vi "SGL to String Exchange.vi"(2 "SGL In":sgl, 3 "4字节字符串":string="C{™š") -> (0 "4字节字符串":string, 1 "IEE754Floatout":sgl format="%#_5f")   [LabVIEW 2015]
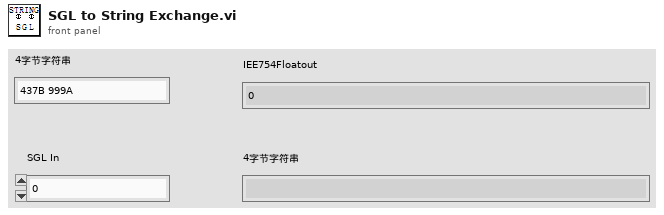
[diagram p1: front panel]
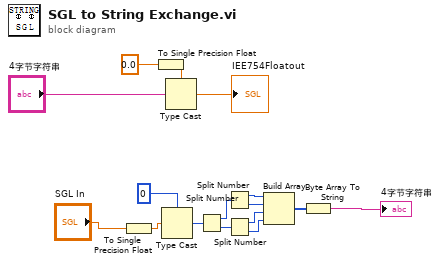
[diagram p0: block diagram]
diagram:
  n1 = To Single Precision Float(number="SGL In") -> (single precision float=w1:sgl)
  n2 = To Single Precision Float(number=sgl 0.0) -> (single precision float=w3:sgl)
  n3 = Type Cast(type=0, x=w1) -> (*(type *) &x=w12:i32)
  n4 = Type Cast(type=w3, x="4字节字符串") -> (*(type *) &x=→"IEE754Floatout":sgl)
  n5 = Split Number(x=w12) -> (hi(x)=w11:u16, lo(x)=w10:u16)
  n6 = Split Number(x=w11) -> (hi(x)=w9:u8, lo(x)=w8:u8)
  n7 = Split Number(x=w10) -> (hi(x)=w7:u8, lo(x)=w6:u8)
  n8 = Build Array(w9, w8, w7, w6) -> (w5:u8[])
  n9 = Byte Array To String(unsigned byte array=w5) -> (string=→"4字节字符串":string)
